vi "xxDbl Array_Linearize NAN values.vi"(10 "Digital":bool, 11 "Dbl Array":dbl[](array[numeric])) -> (2 "Success Out":bool=TRUE, 3 "Dbl Array Out":dbl[](array[numeric]))   [LabVIEW 2020]
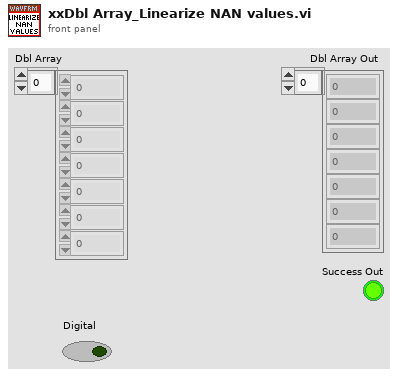
[diagram p1: front panel]
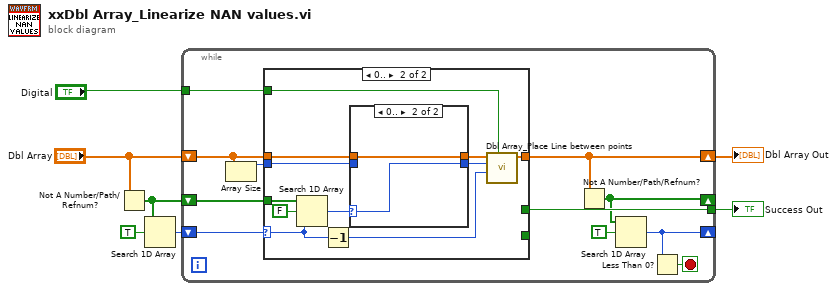
[diagram p0: block diagram]
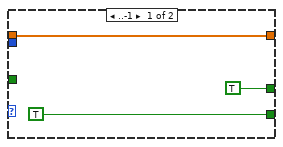
[diagram p2: hidden frame]
diagram:
  n1 = Not A Number/Path/Refnum?(number/path/refnum="Dbl Array") -> (NaN/Path/Refnum?=w3:bool[])
  n2 = Search 1D Array(1D array=w3, element=TRUE) -> (index of element=w2:i32)  [unwired: 1 in]
  n3 = while {
    shift-right: [w12] -> w7
    shift-left: "Dbl Array" -> [w17]
    tunnel: [w18] -> w6
    shift-right: [w10] -> _
    shift-left: w3 -> [w15]
    shift-right: [w9] -> _
    shift-left: w2 -> [w14]
    tunnel: "Digital" -> [w8]
    stop <- w13 stop-if-true
    n4 = Array Size(array=w17) -> (size(s)=w16:i32)
    n5 = case shown="0.." w14 {
      selector: w14 -> [_ w26]
      tunnel: w17 -> [w20 w29]
      tunnel: [TRUE _] -> _
      tunnel: w15 -> [_ w32]
      tunnel: [TRUE _] -> w18
      tunnel: [w20 w27] -> w12
      tunnel: w16 -> [_ w24]
      tunnel: w8 -> [_ w22]
      frame ..-1 {
      }
      frame 0.. {
        n6 = Search 1D Array(1D array=w32, element=FALSE, start index (0)=w26) -> (index of element=w30:i32)
        n7 = Decrement(x=w26) -> (x-1=w23:i32)
        n8 = case shown="0.." w30 {
          selector: w30 -> [_ w35]
          tunnel: w29 -> [w34 w36]
          tunnel: [w34 w36] -> w28
          tunnel: [w33 w35] -> w25
          tunnel: w24 -> [w33 _]
          frame ..-1 {
          }
          frame 0.. {
          }
        }
        n9 = call "Dbl Array_Place Line between points.vi"("Digital"=w22, "Second Index"=w23, "First Index"=w25, "Dbl Array"=w28) -> ("Dbl Array Out"=w27:dbl[])  [unwired: 7 in]
      }
    }
    n10 = Not A Number/Path/Refnum?(number/path/refnum=w12) -> (NaN/Path/Refnum?=w10:bool[])
    n11 = Search 1D Array(1D array=w10, element=TRUE) -> (index of element=w9:i32)  [unwired: 1 in]
    n12 = Less Than 0?(x=w9) -> (x < 0?=w13:bool)
  }
  "Dbl Array Out" <- w7
  "Success Out" <- w6
